vi "Sensors_Alicat.vi"() -> ()   [LabVIEW 2017]
uses:
  Global.vi
panel:
  out "Ar-m' calculated":dbl[unit]=-0.48838499999999996 format="%#_3f"
  out "file size TDMS":dbl=3.064453125
  out "output cluster":cluster{"Array of Waveform":waveform(dbl)[]}={"Array of Waveform"=[{"t0"=timestamp(0 s since 1904-01-01), "dt"=1.0, "Y"=[14.5], "attributes"=variant("Alicat_unit"=variant(string "PSIA"), "NI_ChannelName"=variant(string "Absolute Pressure_O2"), "NI_UnitDescription"=variant(string "psi"))}, {"t0"=timestamp(0 s since 1904-01-01), "dt"=1.0, "Y"=[28.43], "attributes"=variant("Alicat_unit"=variant(string "°C"), "NI_ChannelName"=variant(string "Temperature_O2"), "NI_UnitDescription"=variant(string "degC"))}, {"t0"=timestamp(0 s since 1904-01-01), "dt"=1.0, "Y"=[-0.3], "attributes"=variant("Alicat_unit"=variant(string "LPM"), "NI_ChannelName"=variant(string "Volumetric Flow_O2"), "NI_UnitDescription"=variant(string "l/min"))}, {"t0"=timestamp(0 s since 1904-01-01), "dt"=1.0, "Y"=[-0.3], "attributes"=variant("Alicat_unit"=variant(string "SLPM"), "NI_ChannelName"=variant(string "Mass Flow_O2"), "NI_UnitDescription"=variant(string "kg/min"))}, {"t0"=timestamp(0 s since 1904-01-01), "dt"=1.0, "Y"=[14.56], "attributes"=variant("Alicat_unit"=variant(string "PSIA"), "NI_ChannelName"=variant(string "Absolute Pressure_Ar"), "NI_UnitDescription"=variant(string "psi"))}, {"t0"=timestamp(0 s since 1904-01-01), "dt"=1.0, "Y"=[28.11], "attributes"=variant("Alicat_unit"=variant(string "°C"), "NI_ChannelName"=variant(string "Temperature_Ar"), "NI_UnitDescription"=variant(string "degC"))}, {"t0"=timestamp(0 s since 1904-01-01), "dt"=1.0, "Y"=[0.01], "attributes"=variant("Alicat_unit"=variant(string "LPM"), "NI_ChannelName"=variant(string "Volumetric Flow_Ar"), "NI_UnitDescription"=variant(string "l/min"))}, {"t0"=timestamp(0 s since 1904-01-01), "dt"=1.0, "Y"=[0.01], "attributes"=variant("Alicat_unit"=variant(string "SLPM"), "NI_ChannelName"=variant(string "Mass Flow_Ar"), "NI_UnitDescription"=variant(string "kg/min"))}]}
  out "F-m'":dbl
  out "O2 Volumetric Flow":dbl(knob)=0.01 scale=0.0..450.0 scale format="%#_4g"
  out "O2 Temp":dbl(slide)=28.11 scale=0.0..100.0
  out "O2 Pressure":dbl[unit](knob)=14.56 scale=0.0..450.0 scale format="%#_4g"
  out "O2 Mass flow":dbl[unit](knob)=0.01 scale=0.0..450.0 scale format="%#_4g"
  out "O2 Fuel Ratio":dbl(knob)=inf scale=0.0..6.0
  out "O2-m' calculated":dbl[unit]=0.01302 format="%#_3f"
  out "Ar volumetric Flow":dbl[unit](knob)=-0.3 scale=0.0..450.0 scale format="%#_4g"
  out "Ar Temp":dbl(slide)=28.43 scale=0.0..100.0
  out "Ar-Pressure":dbl[unit](knob)=14.5 scale=0.0..450.0 scale format="%#_4g"
  out "Ar Mass flow":dbl[unit](knob)=-0.3 scale=0.0..450.0 scale format="%#_4g"
  out "TDMS file out":refnum<k34>
  out "TDMS error out":errorcluster
  in  "Save Data TDMS":bool=TRUE
  in  "Stop":bool
  in  "Tab Control":enum32{"File", "Setup"}(tab)
  in  "base path":path=path "E:/Tests"
  out "file path":path=path "E:/Tests/2018-05-14/Run 1_Alicat.tdms"
  in  "Filename":string="Run 1_Alicat"
  in  "AR [ B-19200-COM8]":T1={" ID"="A", "Baud "=enum."19200", "VISA Sesssion In"="COM17"}
  in  "O2 [ A-19200-COM7]":T2={" ID"="B", "Baud"=enum."19200", "VISA Sesssion In"="COM14"}
  in  "Minimum time between \nreadings [ms]":u32=100
  # "Grabs fuel rate from sensors VI if it is running"
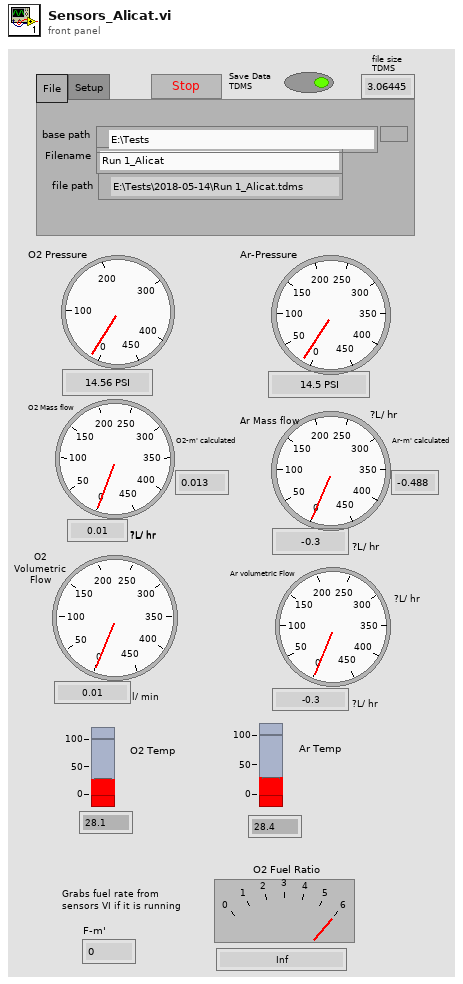
[diagram p1: front panel]
types:
  T1 = cluster{" ID":string, "Baud ":enum8{"2400", "9600", "19200", "38400", "57600", "115200", "Unknown"}, "VISA Sesssion In":refnum<visa-resource-name>}
  T2 = cluster{" ID":string, "Baud":enum8{"2400", "9600", "19200", "38400", "57600", "115200", "Unknown"}, "VISA Sesssion In":refnum<visa-resource-name>}
  T3 = cluster{"Absolute Pressure":bool, "Gauge/Diff. Pressure":bool, "Barometric Pressure":bool, "Temperature":bool, "Volumetric":bool, "Mass":bool, "Setpoint":bool, "Valve Drive":bool, "Totalizer":bool, "Totalizer Timer":bool, "Totalizer Average Flow":bool, "Totalizer Peak Flow":bool, "Gas Selected":bool, "Tot. Timer Format":u16}
  T4 = cluster{"Abs. Pressure":string, "Gauge/Diff. Press.":string, "Barometric Press.":string, "Temperature":string, "Volume":string, "Mass":string, "Setpoint":string, "Valve Drive":string, "Totalizer":string, "Tot. Timer":string, "Tot. Avg. Flow":string, "Tot. Peak Flow":string}
  T5 = cluster{"Absolute Pressure":dbl, "Gauge/Diff. Pressure":dbl, "Barometric Pressure":dbl, "Temperature":dbl, "Volumetric Flow":dbl, "Mass Flow":dbl, "Setpoint":dbl, "Valve Drive":dbl, "Totalizer":dbl, "[hr]":dbl, "[min]":dbl, "[sec]":dbl, "Totalizer Average Flow":dbl, "Totalizer Peak Flow":dbl, "Gas selected":string}
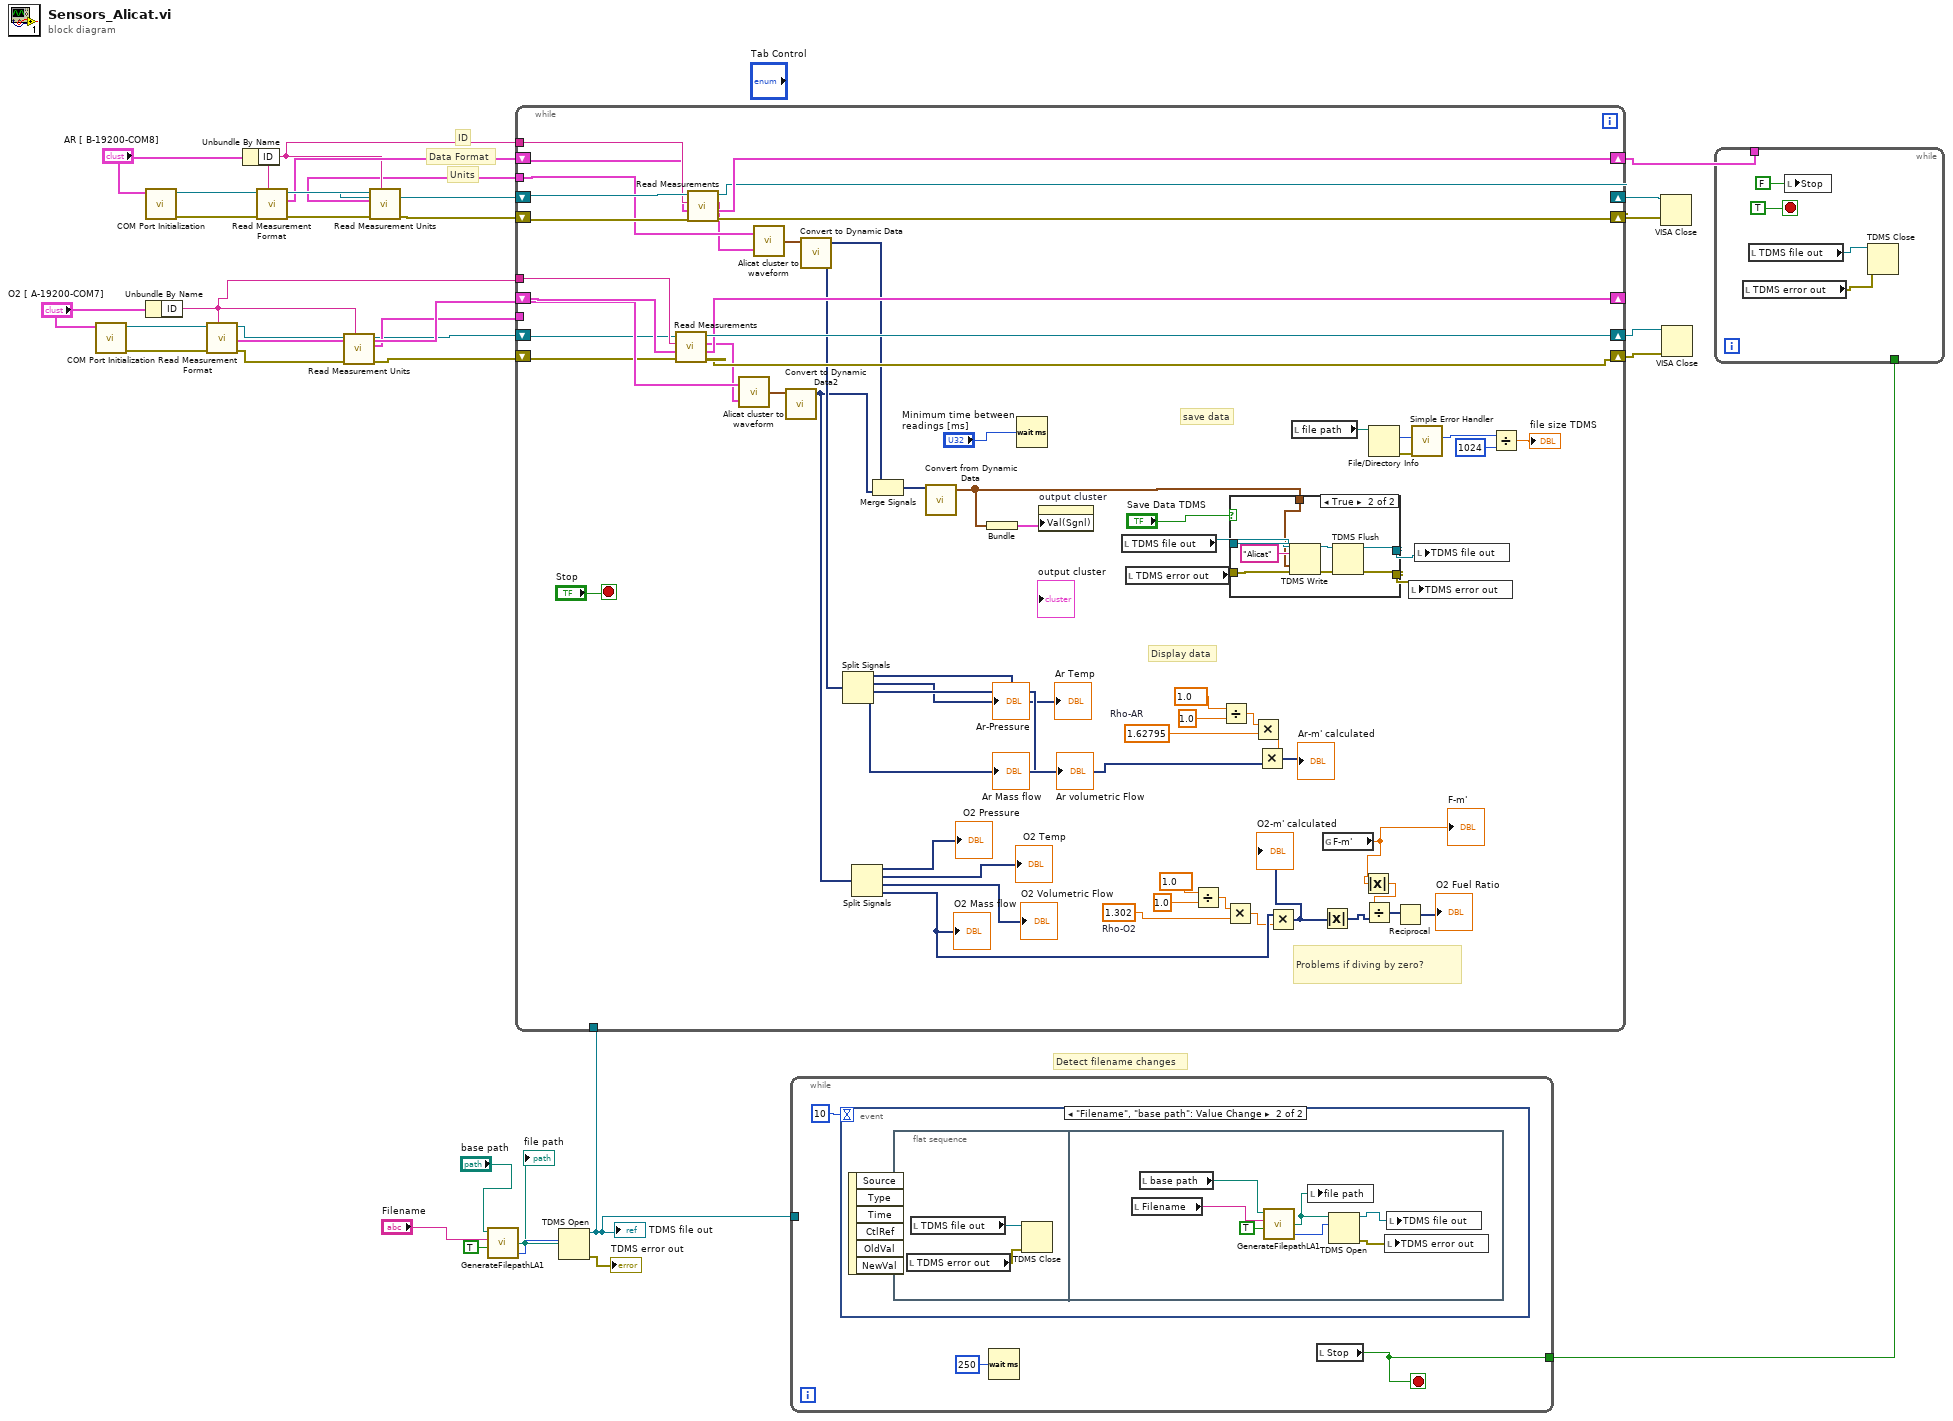
[diagram p0: block diagram]
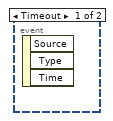
[diagram p3: hidden frame]
diagram:
  # "Units"
  # "Data Format"
  # "ID"
  # "Detect filename changes"
  n1 = call "COM Port Initialization.vi"("Communication Settings"="O2 [ A-19200-COM7]") -> ("error out"=w19:errorcluster, "VISA Session Out"=w18:refnum<visa-resource-name>)  [unwired: 9 in]
  n2 = call "COM Port Initialization.vi"("Communication Settings"="AR [ B-19200-COM8]") -> ("error out"=w20:errorcluster, "VISA Session Out"=w21:refnum<visa-resource-name>)  [unwired: 9 in]
  n3 = Unbundle By Name("O2 [ A-19200-COM7]") -> ("ID"=w8:string)
  n4 = call "Read Measurement Format.vi"("Unit ID (A)"=w8, "error in"=w19, "VISA Session In"=w18) -> ("error out"=w27:errorcluster, "Data Frame Format"=w12:T3, "VISA Session Out"=w26:refnum<visa-resource-name>)  [unwired: 6 in]
  n5 = Unbundle By Name("AR [ B-19200-COM8]") -> ("ID"=w10:string)
  n6 = call "Read Measurement Format.vi"("Unit ID (A)"=w10, "error in"=w20, "VISA Session In"=w21) -> ("error out"=w25:errorcluster, "Data Frame Format"=w15:T3, "VISA Session Out"=w24:refnum<visa-resource-name>)  [unwired: 6 in]
  n7 = call "Read Measurement Units.vi"("Unit ID (A)"=w8, "error in"=w27, "VISA Session In"=w26) -> ("error out"=w5:errorcluster, "Measurement Units"=w11:T4, "VISA Session Out"=w6:refnum<visa-resource-name>)  [unwired: 5 in, 1 out]
  n8 = call "Read Measurement Units.vi"("Unit ID (A)"=w10, "error in"=w25, "VISA Session In"=w24) -> ("error out"=w16:errorcluster, "Measurement Units"=w9:T4, "VISA Session Out"=w17:refnum<visa-resource-name>)  [unwired: 5 in, 1 out]
  n9 = call "GenerateFilepathLA1.vi"("Auto Date folder"=TRUE, "Filename"="Filename", "base path"="base path") -> ("Numeric"=w32:i32, "file path"=w31:path)  [unwired: 1 in, 1 out]
  "file path" <- w31
  n10 = TDMS Open(10:w32, 11:w31) -> (0:→"TDMS error out":errorcluster, 3:w14:refnum<k34>)  [unwired: 5 in]
  "TDMS file out" <- w14
  n11 = while {
    shift-right: [w95] -> w33
    shift-left: w15 -> [w87]
    tunnel: w14 -> [_]
    tunnel: w11 -> [w86]
    tunnel: w10 -> [w89]
    tunnel: w9 -> [w88]
    tunnel: w8 -> [w85]
    shift-right: [w84] -> w4
    shift-left: w16 -> [w94]
    shift-right: [w91] -> w7
    shift-left: w17 -> [w92]
    shift-right: [w79] -> _
    shift-left: w12 -> [w90]
    shift-right: [w80] -> w2
    shift-left: w5 -> [w82]
    shift-right: [w81] -> w3
    shift-left: w6 -> [w83]
    stop <- "Stop" stop-if-true
    w64 = dbl[unit] 1.62795  # Rho-AR
    w51 = dbl[unit] 1.302  # Rho-O2
    # "Display data"
    # "save data"
    # "Problems if diving by zero?"
    n12 = call "Read Measurements.vi"("error in"=w82, "Data Frame Format In"=w90, "Unit ID (A)"=w85, "VISA Session In"=w83) -> ("error out"=w80:errorcluster, "Data Frame Format Out"=w79:T3, "Data Cluster"=w72:T5, "VISA Session Out"=w81:refnum<visa-resource-name>)  [unwired: 4 out]
    n13 = call "Read Measurements.vi"("error in"=w94, "Data Frame Format In"=w87, "Unit ID (A)"=w89, "VISA Session In"=w92) -> ("error out"=w84:errorcluster, "Data Frame Format Out"=w95:T3, "Data Cluster"=w70:T5, "VISA Session Out"=w91:refnum<visa-resource-name>)  [unwired: 4 out]
    n14 = call "Alicat cluster to waveform.vi"("Data Cluster in"=w72, "Measurement Units in"=w86) -> ("Array"=w45:waveform(dbl)[])
    n15 = call "Alicat cluster to waveform.vi"("Data Cluster in"=w70, "Measurement Units in"=w88) -> ("Array"=w71:waveform(dbl)[])
    n16 = call "Convert to Dynamic Data2"("Array of Waveforms"=w45) -> ("Dynamic Data Type"=w43:dynamicdata)  [unwired: 3 in]
    n17 = call "Convert to Dynamic Data"("Array of Waveforms"=w71) -> ("Dynamic Data Type"=w44:dynamicdata)  [unwired: 3 in]
    n18 = Split Signals(w44) -> (→"Ar-Pressure":dynamicdata, →"Ar Temp":dynamicdata, →"Ar volumetric Flow":dynamicdata, w68:dynamicdata)  [unwired: 4 in]
    "Ar Mass flow" <- w68
    n19 = Split Signals(w43) -> (→"O2 Pressure":dynamicdata, →"O2 Temp":dynamicdata, →"O2 Volumetric Flow":dynamicdata, w53:dynamicdata)  [unwired: 4 in]
    "O2 Mass flow" <- w53
    n20 = Merge Signals(w44, w43) -> (w42:dynamicdata)
    n21 = call "Convert from Dynamic Data"("Dynamic Data Type"=w42) -> ("Array of Waveform"=w35:waveform(dbl)[])  [unwired: 3 in]
    n22 = Bundle("Array of Waveform"=w35) -> (w34:cluster{"Array of Waveform":waveform(dbl)[]})  [unwired: 1 in]
    n23 = Wait (ms)(milliseconds to wait="Minimum time between \nreadings [ms]") -> ()  [unwired: 1 out]
    n24 = property on="output cluster" class="Clust (strict)"("Val(Sgnl)"=w34) -> ()  [unwired: 2 in, 2 out]
    n25 = local read "TDMS file out"() -> (w76:refnum<k34>)
    n26 = local read "TDMS error out"() -> (w77:errorcluster)
    n27 = Divide(x=dbl[unit] 1.0, y=dbl[unit] 1.0) -> (x/y=w50:dbl)
    n28 = Divide(x=dbl[unit] 1.0, y=dbl[unit] 1.0) -> (x/y=w66:dbl)
    n29 = Multiply(x=w50, y=w51) -> (x*y=w52:dbl[unit])
    n30 = case shown="True" "Save Data TDMS" {
      tunnel: w76 -> [w97 w102]
      tunnel: w77 -> [w96 w100]
      tunnel: [w97 w105] -> w74
      tunnel: [w96 w104] -> w73
      tunnel: w35 -> [_ w98]
      frame False {
      }
      frame True {
        n31 = TDMS Write(0:w102, 5:"Alicat" ("group name in (Untitled)"), 9:w98, 11:w100) -> (4:w101:refnum<k34>, 15:w99:errorcluster)  [unwired: 2 in, 2 out]
        n32 = TDMS Flush(4:w99, 7:w101) -> (0:w104:errorcluster, 3:w105:refnum<k34>)
      }
    }
    n33 = Multiply(x=w66, y=w64) -> (x*y=w67:dbl[unit])
    n34 = Multiply(x=w67, y=w68) -> (x*y=→"Ar-m' calculated":dynamicdata)
    n35 = Multiply(x=w53, y=w52) -> (x*y=w57:dynamicdata)
    "O2-m' calculated" <- w57
    n36 = local read "file path"() -> (w39:path)
    n37 = Absolute Value(x=w57) -> (abs(x)=w58:dynamicdata)
    n38 = global read "Global.vi" "F-m'"() -> (w41:dbl)
    "F-m'" <- w41
    n39 = Absolute Value(x=w41) -> (abs(x)=w56:dbl)
    n40 = Divide(x=w56, y=w58) -> (x/y=w54:dynamicdata)
    n41 = File/Directory Info(path=w39) -> (size=w37:i64, error out=w40:errorcluster)  [unwired: 1 in, 5 out]
    n42 = Reciprocal(x=w54) -> (1/x=→"O2 Fuel Ratio":dynamicdata)
    n43 = local write "TDMS error out"(w73) -> ()
    n44 = call <vilib>:"Simple Error Handler.vi"("error in (no error)"=w40) -> ()  [unwired: 1 in, 8 out]
    n45 = local write "TDMS file out"(w74) -> ()
    n46 = Divide(x=w37, y=i64 1024) -> (x/y=→"file size TDMS":dbl)
  }
  n47 = while {
    tunnel: w14 -> [_]
    tunnel: [w106] -> w1
    stop <- w106 stop-if-true
    n48 = event shown="[1] \"Filename\", \"base path\": Value Change" {
      selector: _ -> [_ _]
      dyn-events: _ -> [_ _]
      timeout: 10 -> [_ _]
      event Timeout {
        n49 = event-data() -> ()  [unwired: 1 in, 3 out]
      }
      event "Filename", "base path": Value Change {
        n50 = event-data() -> ()  [unwired: 1 in, 6 out]
        n51 = flat-sequence {
          frame #0 {
            n52 = local read "TDMS error out"() -> (w110:errorcluster)
            n53 = local read "TDMS file out"() -> (w109:refnum<k34>)
            n54 = TDMS Close(8:w110, 11:w109) -> ()  [unwired: 2 out]
          }
          frame #1 {
            n55 = local read "Filename"() -> (w117:string)
            n56 = local read "base path"() -> (w116:path)
            n57 = call "GenerateFilepathLA1.vi"("Auto Date folder"=TRUE, "Filename"=w117, "base path"=w116) -> ("Numeric"=w113:i32, "file path"=w115:path)  [unwired: 1 in, 1 out]
            n58 = local write "file path"(w115) -> ()
            n59 = TDMS Open(10:w113, 11:w115) -> (0:w111:errorcluster, 3:w112:refnum<k34>)  [unwired: 5 in]
            n60 = local write "TDMS error out"(w111) -> ()
            n61 = local write "TDMS file out"(w112) -> ()
          }
        }
      }
    }
    n62 = Wait (ms)(milliseconds to wait=u32 250) -> ()  [unwired: 1 out]
    n63 = local read "Stop"() -> (w106:bool)
  }
  n64 = VISA Close(VISA resource name=w7, error in (no error)=w4) -> ()  [unwired: 1 out]
  n65 = VISA Close(VISA resource name=w3, error in (no error)=w2) -> ()  [unwired: 1 out]
  n66 = while {
    tunnel: w33 -> [_]
    tunnel: w1 -> [_]
    stop <- TRUE stop-if-true
    n67 = local read "TDMS error out"() -> (w119:errorcluster)
    n68 = local read "TDMS file out"() -> (w118:refnum<k34>)
    n69 = local write "Stop"(FALSE ("stop_vi")) -> ()
    n70 = TDMS Close(8:w119, 11:w118) -> ()  [unwired: 2 out]
  }
